vi "EditOptions.vi"(8 "error in":errorcluster, 11 "TEC editor node in":refnum<class "TEC editor node.lvclass">) -> (0 "error out":errorcluster, 1 "edit options":T1, 2 "subnodes class":T2, 3 "TEC editor node out":refnum<class "TEC editor node.lvclass">)   [LabVIEW 2013, in "TEC editor node.lvclass"]
doc: "This VI Contains the options for the Menu that will be displayed when doing right click on an item\nThe subnodes class configures which nodes can be added to this nodes\nAnd the edit options determine which options are available for the node.\n\nThis configuration is stored in this VI in case some dynamic configuration is required for the menu options or subnodes.\n\nAll VIs must overide this method"
uses:
  TEC editor node.lvclass
  <vilib>/NI/Configuration Framework/Node/SubNodeCluster.ctl
  <vilib>/NI/Configuration Framework/Node/NodeMenuOptions.ctl
  <vilib>/NI/Configuration Framework/Node/NISE_CEF_Node.lvclass
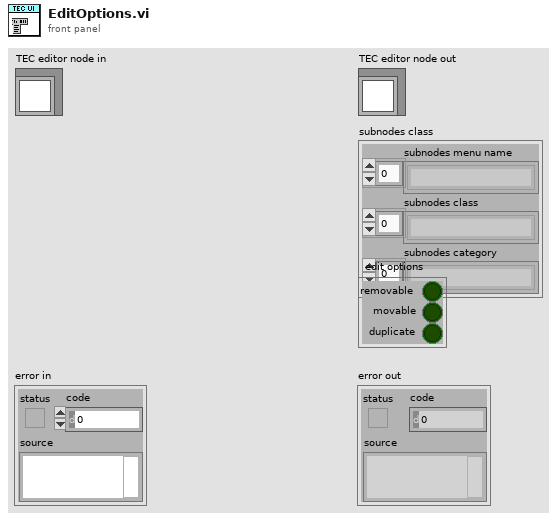
[diagram p1: front panel]
types:
  T1 = typedef "NISE_CEF_Node.lvclass/NodeMenuOptions.ctl" = cluster{"removable":bool, "movable":bool, "duplicate":bool}
  T2 = typedef "NISE_CEF_Node.lvclass/SubNodeCluster.ctl" = cluster{"subnodes menu name":string[], "subnodes class":string[], "subnodes category":string[]}
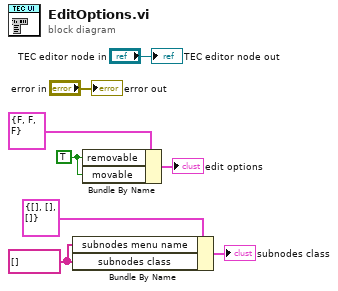
[diagram p0: block diagram]
diagram:
  w3 = TRUE ("removable")
  w4 = string[] [] ("subnodes menu name")
  n1 = Bundle By Name(cluster=T2 {"subnodes menu name"=[], "subnodes class"=[], "subnodes category"=[]} ("subnodes class"), "subnodes menu name"=w4, "subnodes class"=w4) -> (→"subnodes class":T2)
  n2 = Bundle By Name(cluster=T1 {"removable"=FALSE, "movable"=FALSE, "duplicate"=FALSE} ("edit options"), "removable"=w3, "movable"=w3) -> (→"edit options":T1)
  "error out" <- "error in"
  "TEC editor node out" <- "TEC editor node in"
